vi "Structured_Game_Data.vi"() -> ()   [LabVIEW 2017]
uses:
  TypeDef/Game_Data.ctl
panel:
  out "Game Data":T1={"Close  Switch"=enum."Right", "Scale"=enum."Right", "Far Switch"=enum."Right"}
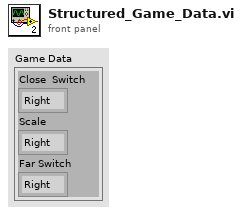
[diagram p1: front panel]
types:
  T1 = typedef "Game_Data.ctl" = cluster{"Close  Switch":enum16{"Left", "Right", "Unknown"}, "Scale":enum16{"Left", "Right", "Unknown"}, "Far Switch":enum16{"Left", "Right", "Unknown"}}
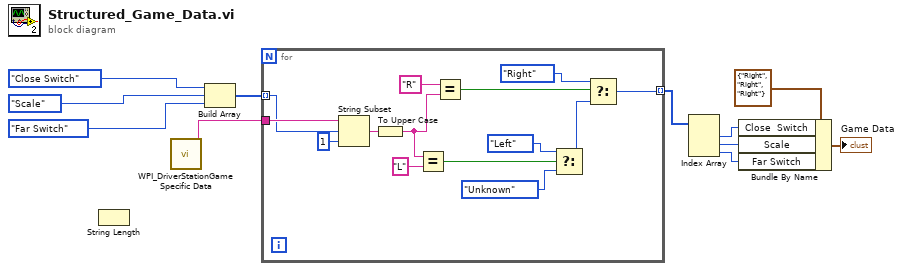
[diagram p0: block diagram]
diagram:
  n1 = String Length() -> ()  [unwired: 1 in, 1 out]
  n2 = call <vilib>:"WPI_DriverStationGame Specific Data.vi"() -> ("Game Specific Data"=w7:string)  [unwired: 11 in]
  n3 = Build Array(enum16{"Close Switch", "Scale", "Far Switch"}."Close Switch" ("Plate Type"), enum16{"Close Switch", "Scale", "Far Switch"}."Scale" ("Plate Type"), enum16{"Close Switch", "Scale", "Far Switch"}."Far Switch" ("Plate Type")) -> (w8:enum16{"Close Switch", "Scale", "Far Switch"}[])
  n4 = for {
    tunnel: w8 -> [w24] mode=indexing
    tunnel: w7 -> [w25]
    tunnel: [w12] -> w5 mode=indexing
    n5 = String Subset(string=w25, offset (0)=w24, length (rest)=1 ("length (rest)")) -> (substring=w22:string)
    n6 = To Upper Case(1:w22) -> (0:w20:string)
    n7 = Equal?(x=w20, y="L") -> (x = y?=w18:bool)
    n8 = Equal?(x="R", y=w20) -> (x = y?=w17:bool)
    n9 = Select(t=enum16{"Left", "Right", "Unknown"}."Left" ("Plate Position"), s=w18, f=enum16{"Left", "Right", "Unknown"}."Unknown" ("Plate Position")) -> (s? t:f=w16:enum16{"Left", "Right", "Unknown"})
    n10 = Select(t=enum16{"Left", "Right", "Unknown"}."Right", s=w17, f=w16) -> (s? t:f=w12:enum16{"Left", "Right", "Unknown"})
  }
  n11 = Index Array(array=w5) -> (element #1=w4:enum16{"Left", "Right", "Unknown"}, element #2=w3:enum16{"Left", "Right", "Unknown"}, element #3=w2:enum16{"Left", "Right", "Unknown"})  [unwired: 3 in]
  n12 = Bundle By Name(cluster=T1 {"Close  Switch"=enum."Right", "Scale"=enum."Right", "Far Switch"=enum."Right"}, "Close  Switch"=w4, "Scale"=w3, "Far Switch"=w2) -> (→"Game Data":T1)
